vi "Get ModAcc Results.vi"(8 "error in (no error)":errorcluster, 11 "niDTS BT INSTR TX in":refnum<class "niDTS BT INSTR TX.lvclass">) -> (0 "error out":errorcluster, 2 "ModaccResults":T1, 3 "niDTS BT INSTR TX out":refnum<class "niDTS BT INSTR TX.lvclass">)   [LabVIEW 2015, in "niDTS BT.lvlib" / "niDTS BT INSTR TX.lvclass"]
uses:
  niDTS BT INSTR TX.lvclass
  Includes/niDTS BT INSTR TX INC ModAcc Result.ctl
  Tests/Tx Test/Includes/niDTS BT Tx Test INC DEVM Results.ctl
  Tests/Tx Test/Includes/niDTS BT Tx Test INC CF Stability Results.ctl
  Tests/Tx Test/Includes/niDTS BT Tx Test INC CFO Resutls.ctl
  Tests/Tx Test/Includes/niDTS BT Tx Test INC Character Results.ctl
  niDTS BT INSTR TX.lvclass/niDTS BT INSTR TX.ctl
  RiviInstDriver/niRfsaBT/Objects/niRfsaBt.lvclass
  niDTS BT.lvlib
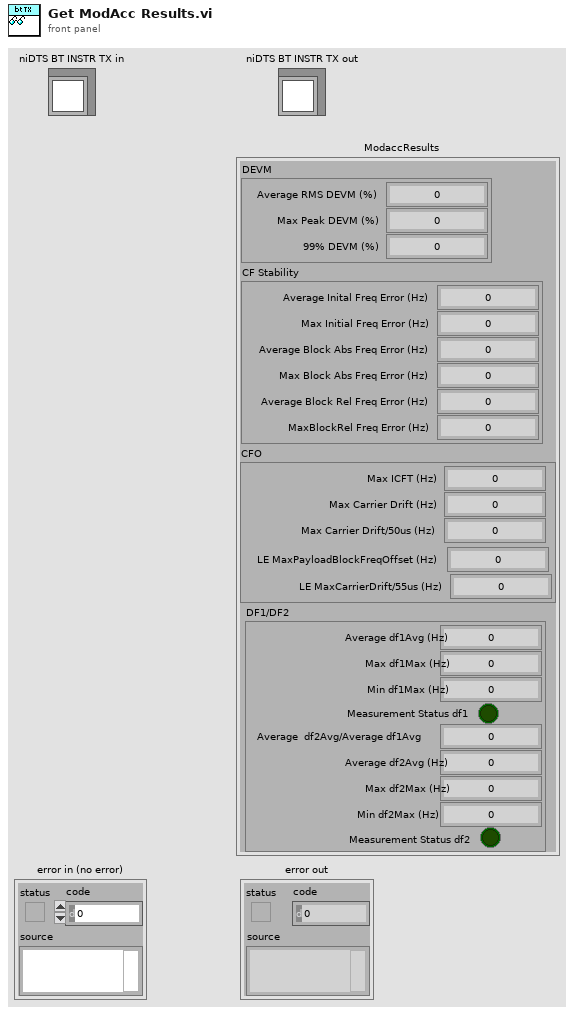
[diagram p1: front panel]
types:
  T1 = typedef "niDTS BT.lvlib/niDTS BT INSTR TX.lvclass/niDTS BT INSTR TX INC ModAcc Result.ctl" = cluster{"DEVM":T2, "CF Stability":T3, "CFO":T4, "DF1/DF2":T5}
  T2 = typedef "niDTS BT.lvlib/niDTS BT Tx Test INC DEVM Results.ctl" = cluster{"Average RMS DEVM (%)":dbl, "Max Peak DEVM (%)":dbl, "99% DEVM (%)":dbl}
  T3 = typedef "niDTS BT.lvlib/niDTS BT Tx Test INC CF Stability Results.ctl" = cluster{"Average Inital Freq Error (Hz)":dbl, "Max Initial Freq Error (Hz)":dbl, "Average Block Abs Freq Error (Hz)":dbl, "Max Block Abs Freq Error (Hz)":dbl, "Average Block Rel Freq Error (Hz)":dbl, "MaxBlockRel Freq Error (Hz)":dbl}
  T4 = typedef "niDTS BT.lvlib/niDTS BT Tx Test INC CFO Resutls.ctl" = cluster{"Max ICFT (Hz)":dbl, "Max Carrier Drift (Hz)":dbl, "Max Carrier Drift/50us (Hz)":dbl, "LE MaxPayloadBlockFreqOffset (Hz)":dbl, "LE MaxCarrierDrift/55us (Hz)":dbl}
  T5 = typedef "niDTS BT.lvlib/niDTS BT Tx Test INC Character Results.ctl" = cluster{"Average df1Avg (Hz)":dbl, "Max df1Max (Hz)":dbl, "Min df1Max (Hz)":dbl, "Measurement Status df1":bool, "Average  df2Avg/Average df1Avg":dbl, "Average df2Avg (Hz)":dbl, "Max df2Max (Hz)":dbl, "Min df2Max (Hz)":dbl, "Measurement Status df2":bool}
  T6 = cluster{"AverageInitialFrequencyError":dbl, "MaxInitialFrequencyError":dbl, "AverageBlockAbsFrequencyError":dbl, "MaxBlockAbsFrequencyError":dbl, "AverageBlockRelFrequencyError":dbl, "MaxBlockRelFrequencyError":dbl}
  T7 = cluster{"AverageRmsDevm":dbl, "MaxPeakDevm":dbl, "99pctDevm":dbl}
  T8 = cluster{"MeasurementStatusDf1":bool, "AverageDf1Avg":dbl, "MaxDf1Max":dbl, "MinDf1Max":dbl, "MeasurementStatusDf2":bool, "AverageDf2Avg":dbl, "MaxDf2Max":dbl, "MinDf2Max":dbl, "AverageDf2avg/AverageDf1avg":dbl}
  T9 = cluster{"IcftMax":dbl, "MaxCarrierDrift":dbl, "MaxCarrierDrift/50us":dbl, "MaxPayloadBlockFreqOffset":dbl, "MaxCarrierDrift/55us":dbl}
  T10 = cluster{"Properties:CFO":cluster{"IcftMax":dbl, "MaxCarrireDrift":dbl, "MaxCarrireDrift/50us":dbl, "MaxPayloadBlockFreqOffset":dbl, "MaxCarrierDrift/55us":dbl}, "Properties:CHARacter":cluster{"MeasurementStatusDf1":bool, "AverageDf1Avg":dbl, "MaxDf1Max":dbl, "MinDf1Max":dbl, "MeasurementStatusDf2":bool, "AverageDf2Avg":dbl, "MaxDf2Max":dbl, "MinDf2Max":dbl, "AverageDf2avg/AverageDf1avg":dbl}, "Properties:CFSTability":cluster{"AverageInitialFrequencyError":dbl, "MaxInitialFrequencyError":dbl, "AverageBlockAbsFrequencyError":dbl, "MaxBlockAbsFrequencyError":dbl, "AverageBlockRelFrequencyError":dbl, "MaxBlockRelFrequencyError":dbl}, "Properties:DEVM":cluster{"AverageRmsDevm":dbl, "MaxPeakDevm":dbl, "99pctDevm":dbl}}
  T11 = typedef "niDTS BT.lvlib/niDTS BT INC Packet Type.ctl" = enum16{"NULL", "POLL", "FHS", "DM1", "DH1", "HV1", "HV2", "HV3", "EV3", "DV", "AUX1", "DM3", "DH3", "EV4", "EV5", "DM5", "DH5", "LE-TP"}
  T12 = typedef "niRfsaBT.lvclass/niRfsaBT INC Handle.ctl" = refnum<data-value>
  T13 = typedef "niDTS BT.lvlib/niDTS BT INC Standard.ctl" = enum16{"BDR", "EDR", "LE-TP"}
  T14 = typedef "niRfsaBt.lvclass/niRfsaBt INC Handle.ctl" = refnum<data-value>
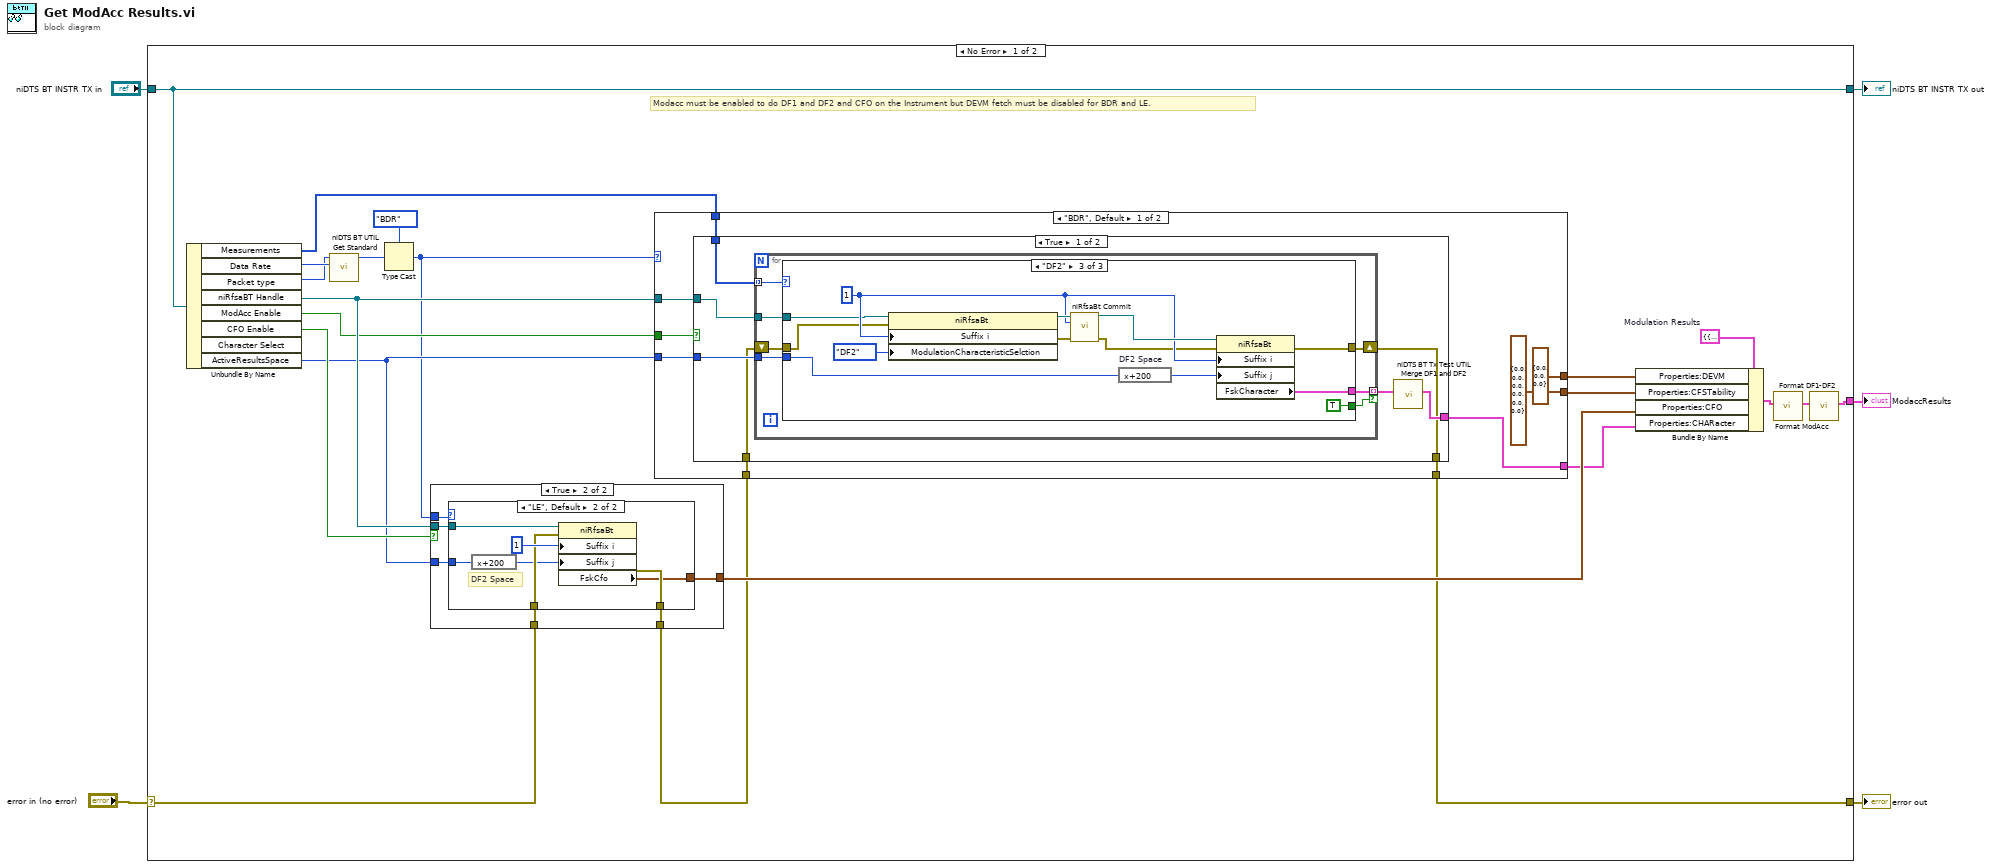
[diagram p0: block diagram]
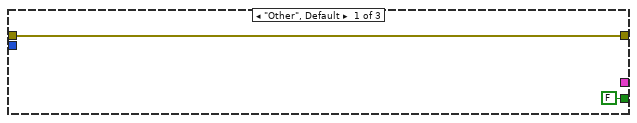
[diagram p2: hidden frame]
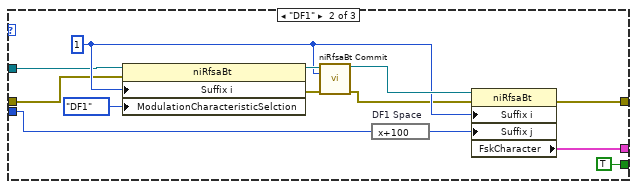
[diagram p3: hidden frame]
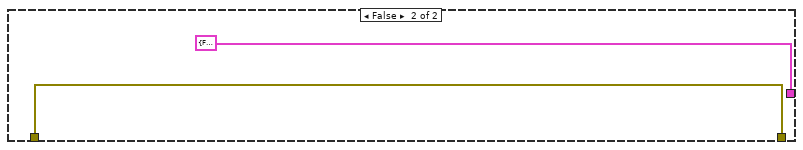
[diagram p4: hidden frame]
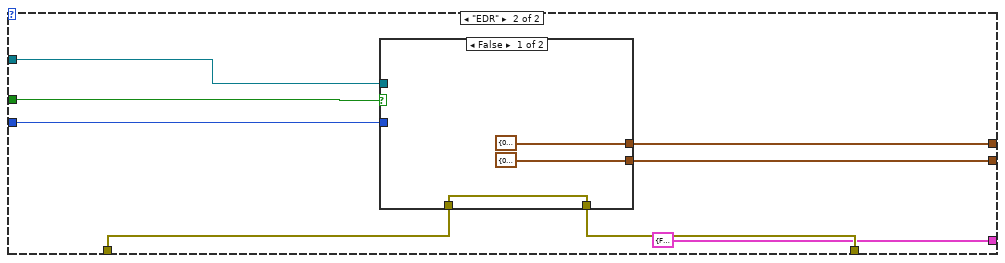
[diagram p5: hidden frame]
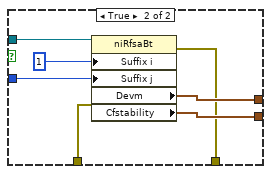
[diagram p6: hidden frame]
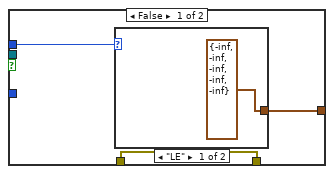
[diagram p7: hidden frame]
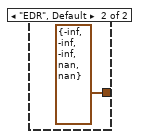
[diagram p8: hidden frame]
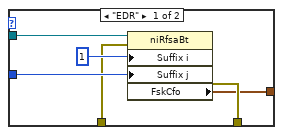
[diagram p9: hidden frame]
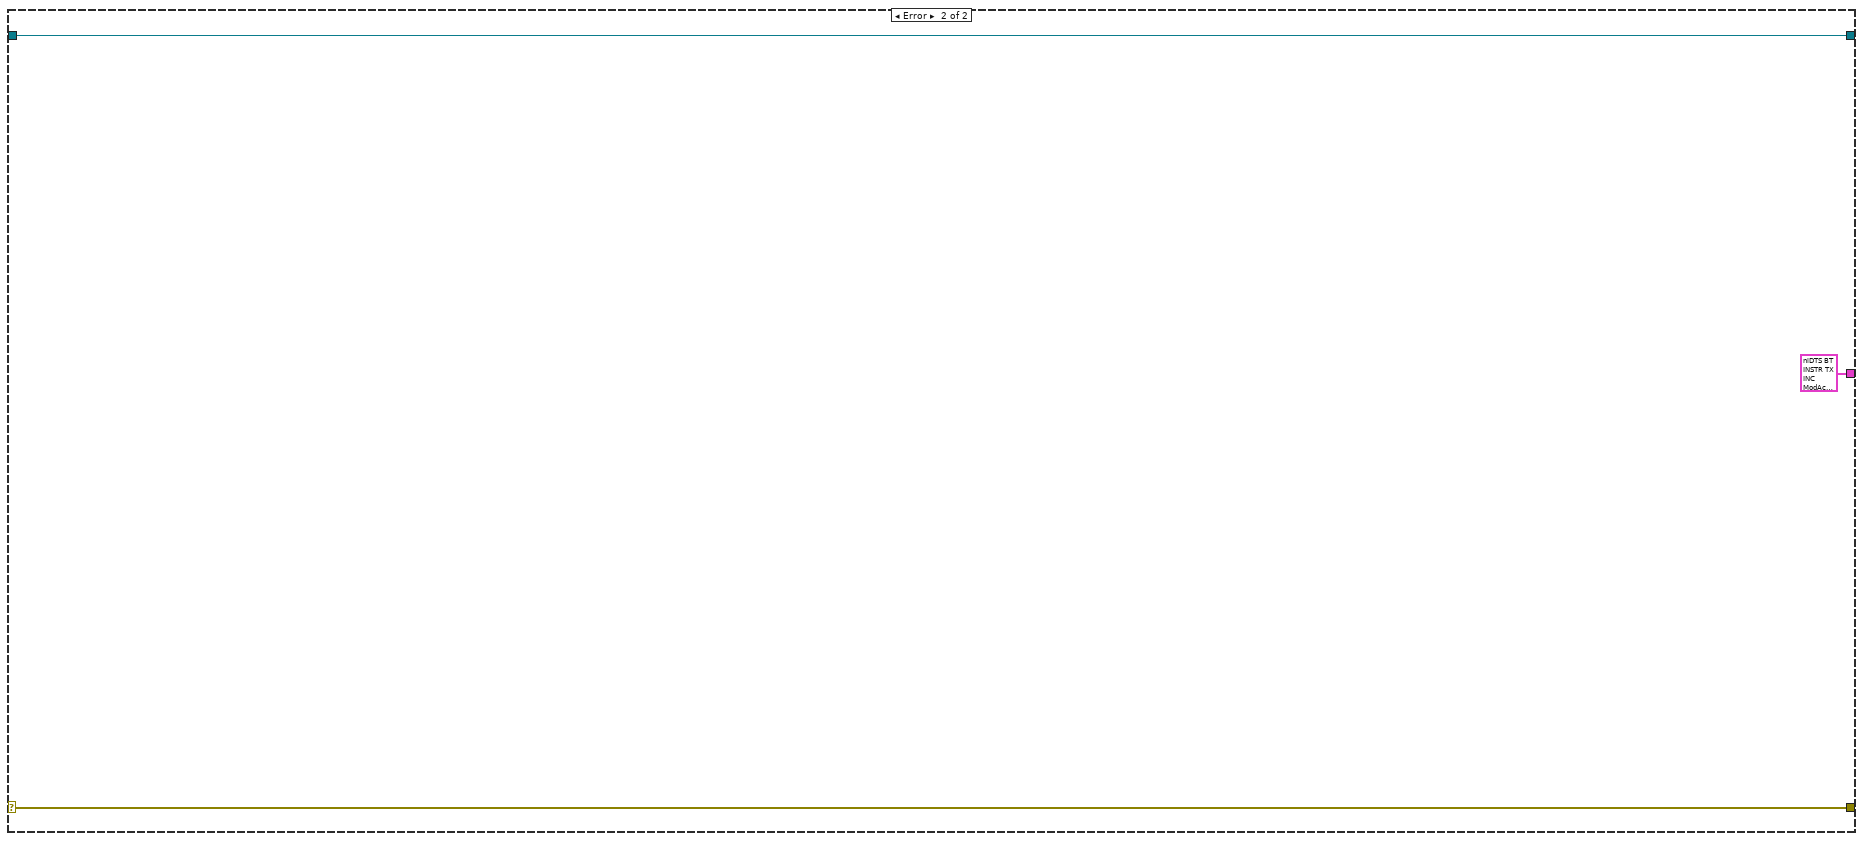
[diagram p10: hidden frame]
diagram:
  n1 = case shown="No Error" "error in (no error)" {
    selector: "error in (no error)" -> [w8 w124]
    tunnel: [w17 w124] -> w2
    tunnel: [w27 w125] -> w3
    tunnel: "niDTS BT INSTR TX in" -> [w27 w125]
    tunnel: [w19 T1 {"DEVM"={"Average RMS DEVM (%)"=0.0, "Max Peak DEVM (%)"=0.0, "99% DEVM (%)"=0.0}, "CF Stability"={"Average Inital Freq Error (Hz)"=0.0, "Max Initial Freq Error (Hz)"=0.0, "Average Block Abs Freq Error (Hz)"=0.0, "Max Block Abs Freq Error (Hz)"=0.0, "Average Block Rel Freq Error (Hz)"=0.0, "MaxBlockRel Freq Error (Hz)"=0.0}, "CFO"={"Max ICFT (Hz)"=0.0, "Max Carrier Drift (Hz)"=0.0, "Max Carrier Drift/50us (Hz)"=0.0, "LE MaxPayloadBlockFreqOffset (Hz)"=0.0, "LE MaxCarrierDrift/55us (Hz)"=0.0}, "DF1/DF2"={"Average df1Avg (Hz)"=0.0, "Max df1Max (Hz)"=0.0, "Min df1Max (Hz)"=0.0, "Measurement Status df1"=FALSE, "Average  df2Avg/Average df1Avg"=0.0, "Average df2Avg (Hz)"=0.0, "Max df2Max (Hz)"=0.0, "Min df2Max (Hz)"=0.0, "Measurement Status df2"=FALSE}} ("output cluster")] -> w1
    frame No Error {
      w11 = T10 {"Properties:CFO"={"IcftMax"=0.0, "MaxCarrireDrift"=0.0, "MaxCarrireDrift/50us"=0.0, "MaxPayloadBlockFreqOffset"=0.0, "MaxCarrierDrift/55us"=0.0}, "Properties:CHARacter"={"MeasurementStatusDf1"=FALSE, "AverageDf1Avg"=0.0, "MaxDf1Max"=0.0, "MinDf1Max"=0.0, "MeasurementStatusDf2"=FALSE, "AverageDf2Avg"=0.0, "MaxDf2Max"=0.0, "MinDf2Max"=0.0, "AverageDf2avg/AverageDf1avg"=0.0}, "Properties:CFSTability"={"AverageInitialFrequencyError"=0.0, "MaxInitialFrequencyError"=0.0, "AverageBlockAbsFrequencyError"=0.0, "MaxBlockAbsFrequencyError"=0.0, "AverageBlockRelFrequencyError"=0.0, "MaxBlockRelFrequencyError"=0.0}, "Properties:DEVM"={"AverageRmsDevm"=0.0, "MaxPeakDevm"=0.0, "99pctDevm"=0.0}}  # Modulation Results
      # "Modacc must be enabled to do DF1 and DF2 and CFO on the Instrument but DEVM fetch must be disabled for BDR and LE."
      n2 = Unbundle By Name(w27) -> ("Measurements"=w6:enum16{"Other", "DF1", "DF2"}[], "Data Rate"=w14:i32, "Packet type"=w13:T11, "niRfsaBT Handle"=w22:T12, "ModAcc Enable"=w10:bool, "CFO Enable"=w24:bool, "ActiveResultsSpace"=w18:u8)  [unwired: 1 out]
      n3 = call "niDTS BT UTIL Get Standard.vi"("Data Rate"=w14, "Packet type"=w13) -> ("BT Standard"=w12:T13)  [unwired: 9 in]
      n4 = Type Cast(type=enum16{"BDR", "EDR", "LE"}."BDR" ("Standard"), x=w12) -> (*(type *) &x=w7:enum16{"BDR", "EDR", "LE"})
      n5 = case shown="True" w24 {
        tunnel: w22 -> [_ w109]
        tunnel: [w100 w105] -> w23
        tunnel: w18 -> [_ w108]
        tunnel: w8 -> [w101 w107]
        tunnel: [w101 w106] -> w16
        tunnel: w7 -> [w99 w104]
        frame False {
          n6 = case shown="\"LE\"" w99 {
            tunnel: [T9 {"IcftMax"=-inf, "MaxCarrierDrift"=-inf, "MaxCarrierDrift/50us"=-inf, "MaxPayloadBlockFreqOffset"=-inf, "MaxCarrierDrift/55us"=-inf} ("Cfo") T9 {"IcftMax"=-inf, "MaxCarrierDrift"=-inf, "MaxCarrierDrift/50us"=-inf, "MaxPayloadBlockFreqOffset"=nan, "MaxCarrierDrift/55us"=nan} ("Cfo")] -> w100
            frame "LE" {
            }
            frame "EDR", Default {
            }
          }
        }
        frame True {
          n7 = case shown="\"LE\", Default" w104 {
            tunnel: w109 -> [w115 w122]
            tunnel: w108 -> [w113 w120]
            tunnel: w107 -> [w112 w119]
            tunnel: [w111 w118] -> w106
            tunnel: [w110 w117] -> w105
            frame "EDR" {
              n8 = property class="niRfsaBt"(reference=w115, error in=w112, "Suffix i"=1 ("Active Channel:Suffix i"), "Suffix j"=w113) -> (error out=w111:errorcluster, "FskCfo"=w110:T9)  [unwired: 1 out]
            }
            frame "LE", Default {
              # "DF2 Space"
              n9 = expression code="x+200"(w120) -> (w116:u8)
              n10 = property class="niRfsaBt"(reference=w122, error in=w119, "Suffix i"=1 ("Active Channel:Suffix i"), "Suffix j"=w116) -> (error out=w118:errorcluster, "FskCfo"=w117:T9)  [unwired: 1 out]
            }
          }
        }
      }
      n11 = case shown="\"BDR\", Default" w7 {
        tunnel: [T7 {"AverageRmsDevm"=0.0, "MaxPeakDevm"=0.0, "99pctDevm"=0.0} ("DEVM") w88] -> w26
        tunnel: [T6 {"AverageInitialFrequencyError"=0.0, "MaxInitialFrequencyError"=0.0, "AverageBlockAbsFrequencyError"=0.0, "MaxBlockAbsFrequencyError"=0.0, "AverageBlockRelFrequencyError"=0.0, "MaxBlockRelFrequencyError"=0.0} ("CFSTability") w87] -> w25
        tunnel: w22 -> [w34 w86]
        tunnel: w18 -> [w33 w85]
        tunnel: [w29 w84] -> w17
        tunnel: w16 -> [w31 w83]
        tunnel: w10 -> [w32 w82]
        tunnel: [w30 T8 {"MeasurementStatusDf1"=FALSE, "AverageDf1Avg"=nan, "MaxDf1Max"=nan, "MinDf1Max"=nan, "MeasurementStatusDf2"=FALSE, "AverageDf2Avg"=nan, "MaxDf2Max"=nan, "MinDf2Max"=nan, "AverageDf2avg/AverageDf1avg"=-inf} ("Properties:CHARacter")] -> w9
        tunnel: w6 -> [w28 _]
        frame "BDR", Default {
          n12 = case shown="True" w32 {
            tunnel: w34 -> [w41 _]
            tunnel: [w43 T8 {"MeasurementStatusDf1"=FALSE, "AverageDf1Avg"=nan, "MaxDf1Max"=nan, "MinDf1Max"=nan, "MeasurementStatusDf2"=FALSE, "AverageDf2Avg"=nan, "MaxDf2Max"=nan, "MinDf2Max"=nan, "AverageDf2avg/AverageDf1avg"=-inf} ("Character")] -> w30
            tunnel: w33 -> [w42 _]
            tunnel: w31 -> [w37 w79]
            tunnel: [w38 w79] -> w29
            tunnel: w28 -> [w40 _]
            frame True {
              n13 = for {
                tunnel: w40 -> [w50] mode=indexing
                tunnel: w41 -> [w49]
                tunnel: w42 -> [w48]
                tunnel: [w47] -> w39 mode=indexing if=w46
                shift-right: [w45] -> w38
                shift-left: w37 -> [w44]
                n14 = case shown="\"DF2\"" w50 {
                  tunnel: w49 -> [_ w58 w71]
                  tunnel: w48 -> [_ w57 w70]
                  tunnel: [_ w56 w69] -> w47
                  tunnel: [FALSE ("MeasurementStatusDf1") TRUE ("MeasurementStatusDf1") TRUE ("MeasurementStatusDf1")] -> w46
                  tunnel: [w51 w54 w67] -> w45
                  tunnel: w44 -> [w51 w53 w66]
                  frame "Other", Default {
                  }
                  frame "DF1" {
                    w60 = 1 ("Active Channel:Suffix i")
                    n15 = property class="niRfsaBt"(reference=w58, error in=w53, "Suffix i"=w60, "ModulationCharacteristicSelction"=enum16{"DF1", "DF2"}."DF1" ("CONFigure:RFSA:BLUetooth:MEASurement:MODulation:FSK:CHARacter:ModulationCharacteristicSelction")) -> (reference out=w64:T12, error out=w62:errorcluster)
                    n16 = call "niRfsaBt Commit.vi"("InstDriver Handle in"=w64, "Instance"=w60, "error in (no error)"=w62) -> ("InstDriver Handle out"=w61:T14, "error out"=w59:errorcluster)  [unwired: 11 in]
                    n17 = expression code="x+100" "DF1 Space"(w57) -> (w65:u8)
                    n18 = property class="niRfsaBt"(reference=w61, error in=w59, "Suffix i"=w60, "Suffix j"=w65) -> (error out=w54:errorcluster, "FskCharacter"=w56:T8)  [unwired: 1 out]
                  }
                  frame "DF2" {
                    w73 = 1 ("Active Channel:Suffix i")
                    n19 = property class="niRfsaBt"(reference=w71, error in=w66, "Suffix i"=w73, "ModulationCharacteristicSelction"=enum16{"DF1", "DF2"}."DF2" ("CONFigure:RFSA:BLUetooth:MEASurement:MODulation:FSK:CHARacter:ModulationCharacteristicSelction")) -> (reference out=w77:T12, error out=w75:errorcluster)
                    n20 = call "niRfsaBt Commit.vi"("InstDriver Handle in"=w77, "Instance"=w73, "error in (no error)"=w75) -> ("InstDriver Handle out"=w74:T14, "error out"=w72:errorcluster)  [unwired: 11 in]
                    n21 = expression code="x+200" "DF2 Space"(w70) -> (w78:u8)
                    n22 = property class="niRfsaBt"(reference=w74, error in=w72, "Suffix i"=w73, "Suffix j"=w78) -> (error out=w67:errorcluster, "FskCharacter"=w69:T8)  [unwired: 1 out]
                  }
                }
              }
              n23 = call "niDTS BT Tx Test UTIL Merge DF1 and DF2.vi"("DF Array"=w39) -> ("DF1 and DF2"=w43:T8)  [unwired: 10 in]
            }
            frame False {
            }
          }
        }
        frame "EDR" {
          n24 = case shown="False" w82 {
            tunnel: w86 -> [_ w98]
            tunnel: [T7 {"AverageRmsDevm"=0.0, "MaxPeakDevm"=0.0, "99pctDevm"=0.0} ("DEVM") w95] -> w88
            tunnel: [T6 {"AverageInitialFrequencyError"=0.0, "MaxInitialFrequencyError"=0.0, "AverageBlockAbsFrequencyError"=0.0, "MaxBlockAbsFrequencyError"=0.0, "AverageBlockRelFrequencyError"=0.0, "MaxBlockRelFrequencyError"=0.0} ("CFSTability") w96] -> w87
            tunnel: w85 -> [_ w94]
            tunnel: w83 -> [w89 w93]
            tunnel: [w89 w92] -> w84
            frame False {
            }
            frame True {
              n25 = property class="niRfsaBt"(reference=w98, error in=w93, "Suffix i"=1 ("Active Channel:Suffix i"), "Suffix j"=w94) -> (error out=w92:errorcluster, "Devm"=w95:T7, "Cfstability"=w96:T6)  [unwired: 1 out]
            }
          }
        }
      }
      n26 = Bundle By Name(cluster=w11, "Properties:DEVM"=w26, "Properties:CFSTability"=w25, "Properties:CFO"=w23, "Properties:CHARacter"=w9) -> (w21:T10)
      n27 = call "Format ModAcc.vi"("Modulation Results"=w21) -> ("Modulation Results"=w20:T1)  [unwired: 10 in]
      n28 = call "Format DF1-DF2.vi"("Resutls In"=w20) -> ("Results Out"=w19:T1)  [unwired: 10 in]
    }
    frame Error {
    }
  }
  "error out" <- w2
  "niDTS BT INSTR TX out" <- w3
  "ModaccResults" <- w1
